vi "Círculos de Mohr.vi"(1 "R":dbl, 2 "P":dbl, 3 "Sx":dbl) -> (0 "Círculo de Mohr":cluster{"Array":dbl[], "Array":dbl[]}[](array[cluster]))   [LabVIEW 2018]
uses:
  <vilib>/Analysis/1siggen.llb/Ramp Pattern by Samples.vi
  <vilib>/Analysis/NI_AALBase.lvlib
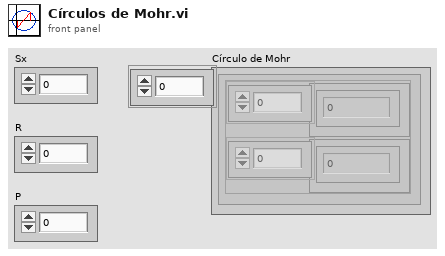
[diagram p1: front panel]
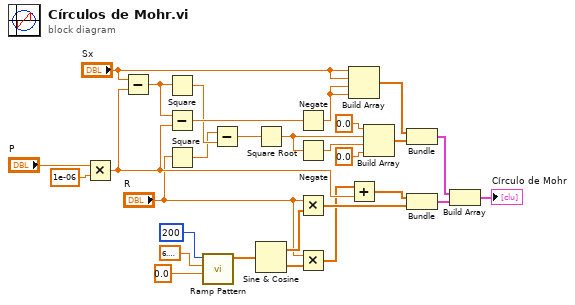
[diagram p0: block diagram]
diagram:
  n1 = Multiply(x="P", y=1e-06) -> (x*y=w29:dbl)
  n2 = Subtract(x="Sx", y=w29) -> (x-y=w24:dbl)
  n3 = Square(x=w24) -> (x^2=w13:dbl)
  n4 = Subtract(x=w24, y=w29) -> (x-y=w25:dbl)
  n5 = Square(x="R") -> (x^2=w12:dbl)
  n6 = call-poly <vilib>:"Ramp Pattern.vi"("start"=0.0, "end"=6.283185307179586, "samples"=200) -> ("Ramp Pattern"=w6:dbl[])  [unwired: 7 in, 1 out]
  n7 = Subtract(x=w12, y=w13) -> (x-y=w22:dbl)
  n8 = Square Root(x=w22) -> (sqrt(x)=w15:dbl)
  n9 = Sine & Cosine(0:w6) -> (1:w9:dbl[], 2:w7:dbl[])
  n10 = Negate(x=w25) -> (-x=w26:dbl)
  n11 = Negate(x=w15) -> (-x=w16:dbl)
  n12 = Multiply(x="R", y=w9) -> (x*y=w11:dbl[])
  n13 = Multiply(x="R", y=w7) -> (x*y=w8:dbl[])
  n14 = Build Array("Sx", "Sx", w26, w26) -> (w27:dbl[])
  n15 = Add(x=w8, y=w29) -> (x+y=w10:dbl[])
  n16 = Build Array(0.0 ("element"), w15, w16, 0.0 ("element")) -> (w21:dbl[])
  n17 = Bundle(w27, w21) -> (w18:cluster{dbl[], dbl[]})  [unwired: 1 in]
  n18 = Bundle(w10, w11) -> (w19:cluster{dbl[], dbl[]})  [unwired: 1 in]
  n19 = Build Array(w18, w19) -> (→"Círculo de Mohr":cluster{dbl[], dbl[]}[])
